vi "Update Save Path.vi"(10 "Process Name":string, 11 "Current Path":path) -> (3 "Updated Path":path)   [LabVIEW 2020, in "Process Generation.lvlib" / "New Class Dialog.lvclass"]
uses:
  New Class Dialog.lvclass
  New Class Dialog.lvclass/New Class Dialog.ctl
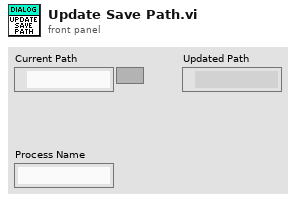
[diagram p1: front panel]
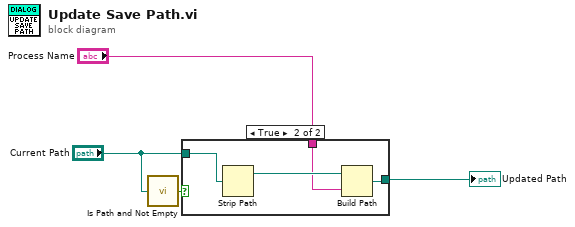
[diagram p0: block diagram]
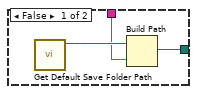
[diagram p2: hidden frame]
diagram:
  n1 = call <vilib>:"Is Path and Not Empty.vi"("path"="Current Path") -> ("Is Path and Not Empty?"=w3:bool)  [unwired: 4 in]
  n2 = case shown="True" w3 {
    tunnel: "Current Path" -> [_ w11]
    tunnel: "Process Name" -> [w6 w9]
    tunnel: [w5 w8] -> w4
    frame False {
      n3 = call "Get Default Save Folder Path.vi"() -> ("Path"=w7:path)  [unwired: 11 in]
      n4 = Build Path(base path=w7, name or relative path=w6) -> (appended path=w5:path)
    }
    frame True {
      n5 = Strip Path(path=w11) -> (stripped path=w10:path)  [unwired: 1 out]
      n6 = Build Path(base path=w10, name or relative path=w9) -> (appended path=w8:path)
    }
  }
  "Updated Path" <- w4
